vi "loadHTOutcounterFixHeader.vi"() -> ()   [LabVIEW 2012]
uses:
  <vilib>/addons/database/Connection.llb/DB Tools Open Connec (Path).vi
  <vilib>/Utility/file.llb/Read From Spreadsheet File (string).vi
  <vilib>/addons/database/Connection.llb/Conn Execute.vi
  <vilib>/addons/database/Recordset.llb/Rec Fetch Integer Data (R).vi
  <vilib>/addons/database/Recordset.llb/Rec Destroy - Connection.vi
  <vilib>/addons/database/NI_Database_API.lvlib
panel:
  out "before substring":string
  out "x > y?":bool
  out "error out":errorcluster
  in  "file (use dialog)":path=path "C:/temp/ht/MachineState/MachineState.txt"
  out "ToRunSite":string
  out "error out 2":errorcluster
  in  "input cluster":T1
  out "output cluster":T1
  out "SQLDateTime":string
  out "time stamp":timestamp
  out "SQLDateTime 2":string
  out "concatenated string":string
  out "all rows":string[][](array[string])
  out "size(s)":i32[](array[numeric])
  out "output cluster 2":T2
  in  "input cluster 2":T2
  out "before substring 5":string
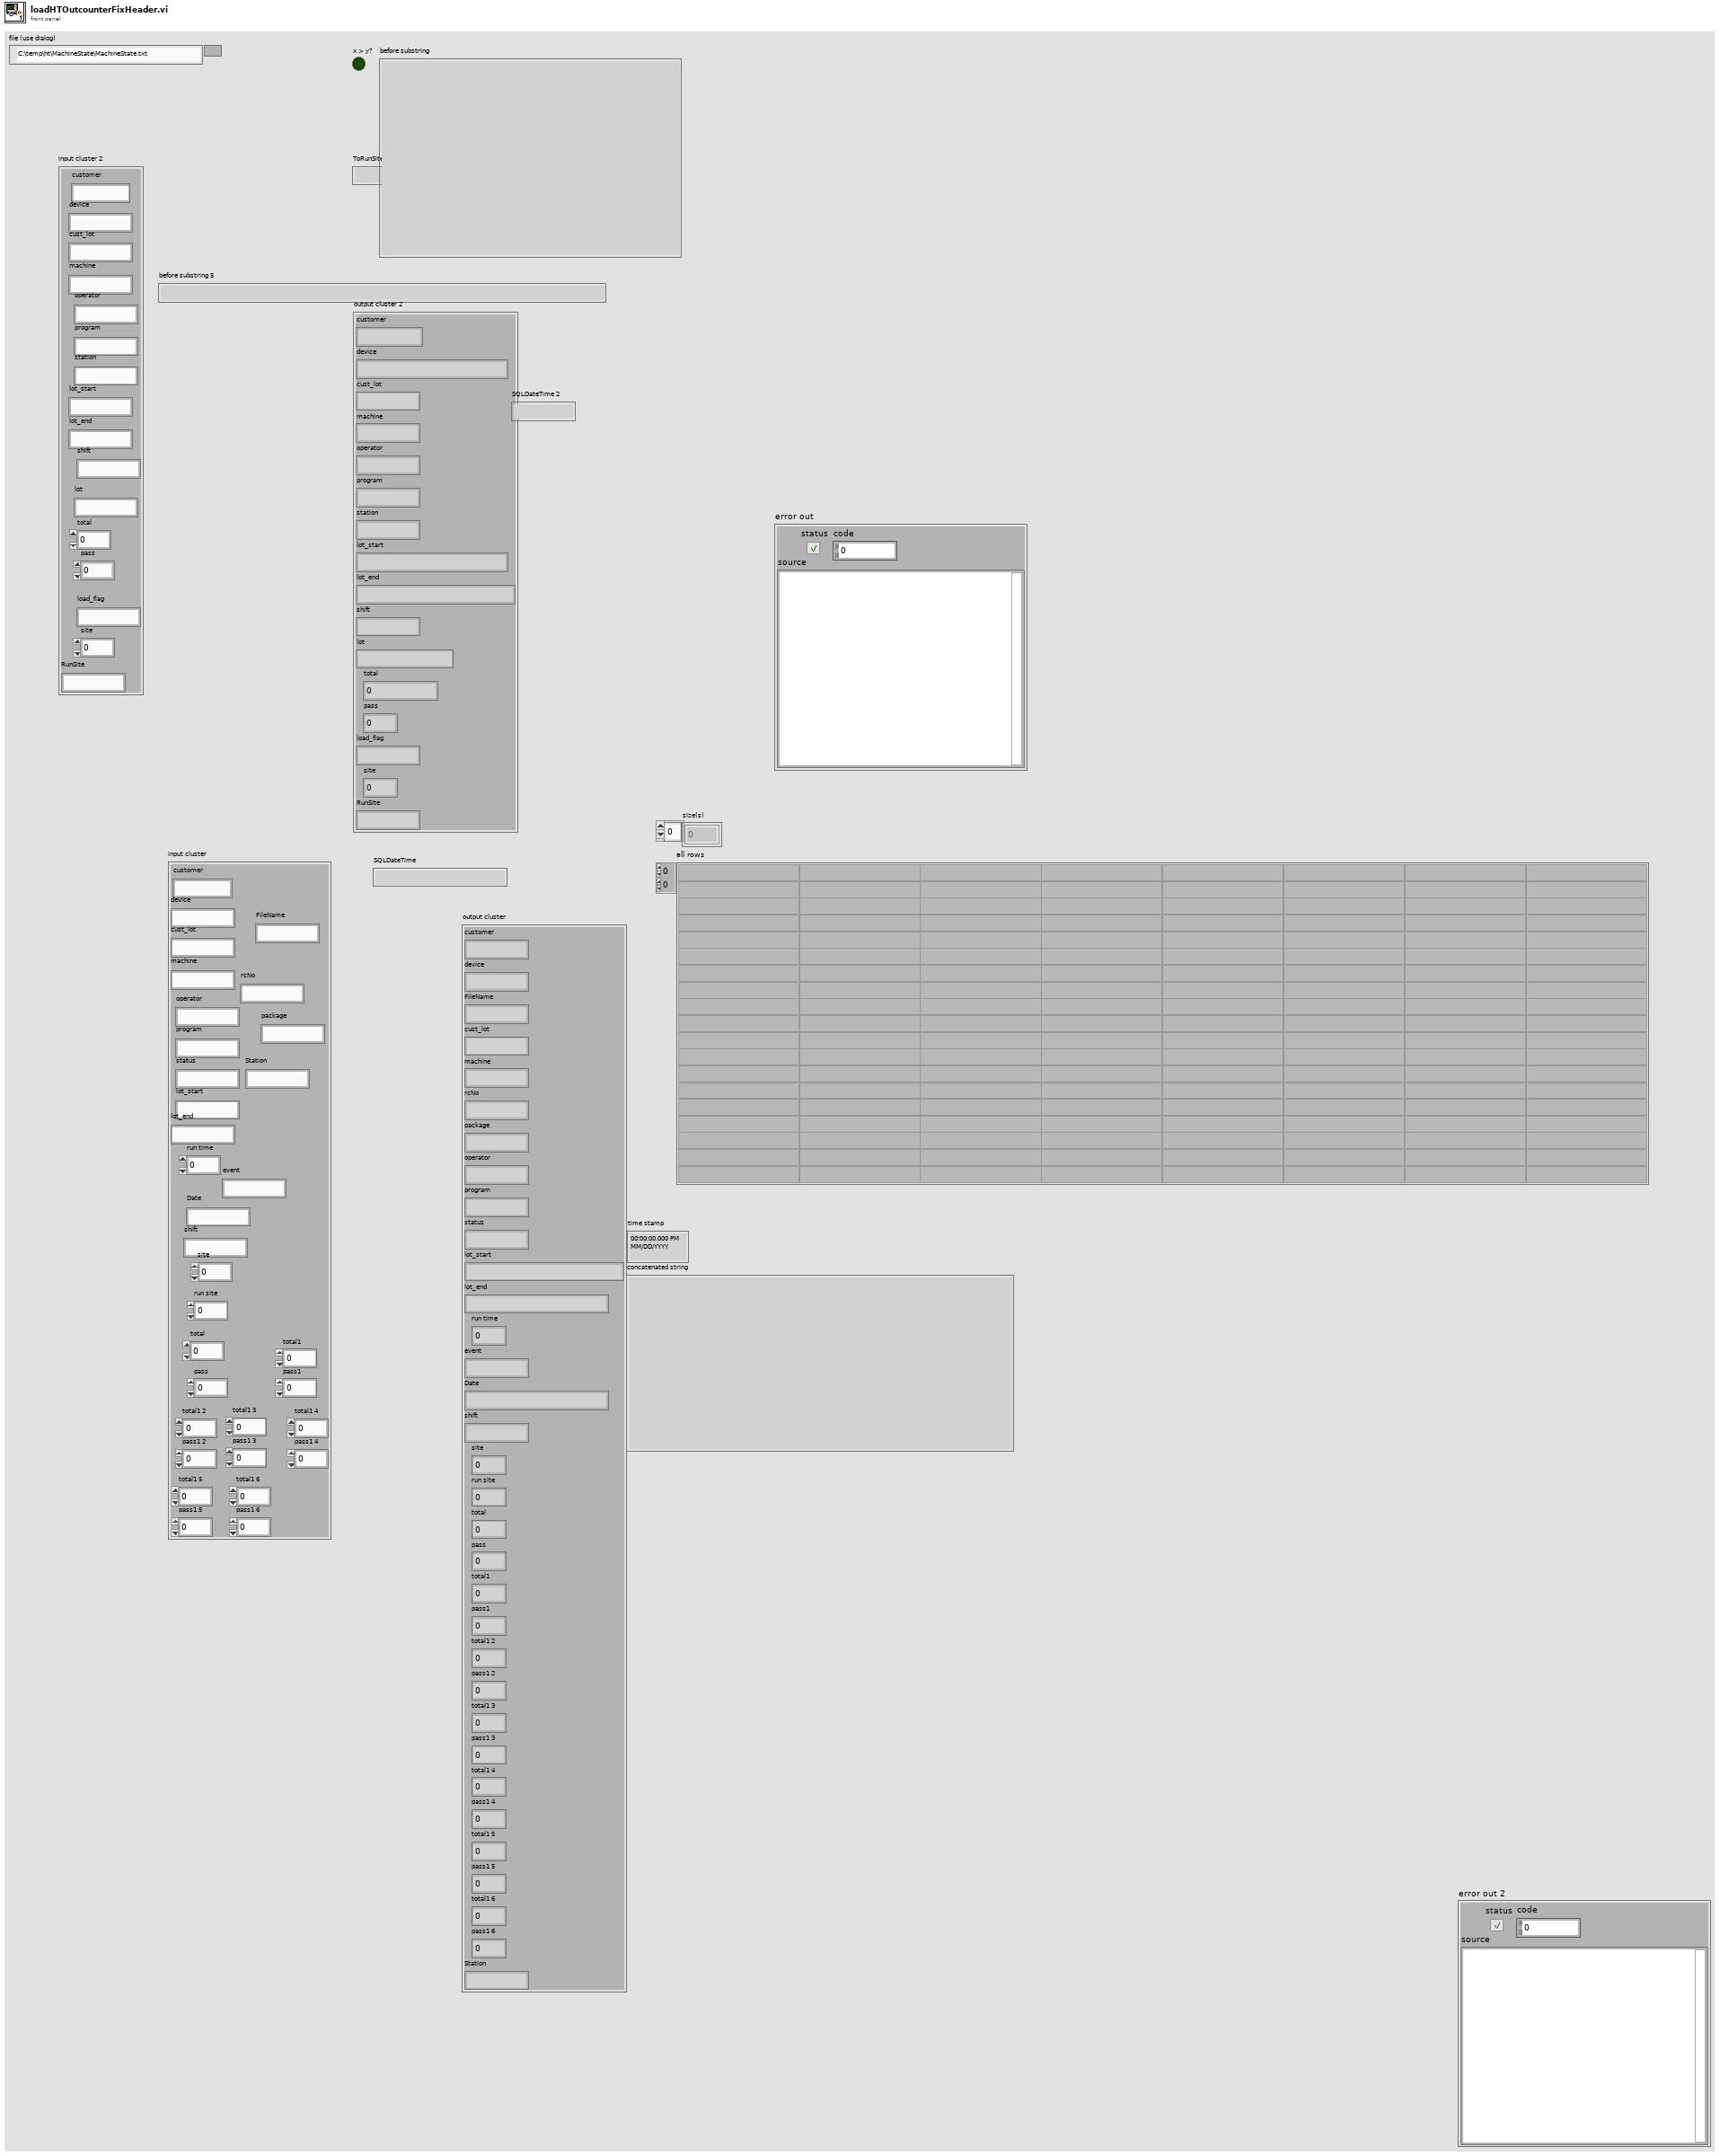
[diagram p1: front panel]
types:
  T1 = cluster{"customer":string, "device":string, "FileName":string, "cust_lot":string, "machine":string, "rcNo":string, "package":string, "operator":string, "program":string, "status":string, "lot_start":string, "lot_end":string, "run time":dbl, "event":string, "Date":string, "shift":string, "site":dbl, "run site ":dbl, "total":dbl, "pass":dbl, "total1":dbl, "pass1":dbl, "total1 2":dbl, "pass1 2":dbl, "total1 3":dbl, "pass1 3":dbl, "total1 4":dbl, "pass1 4":dbl, "total1 5":dbl, "pass1 5":dbl, "total1 6":dbl, "pass1 6":dbl, "Station":string}
  T2 = cluster{"customer":string, "device":string, "cust_lot":string, "machine":string, "operator":string, "program":string, "station":string, "lot_start":string, "lot_end":string, "shift":string, "lot":string, "total":dbl, "pass":dbl, "load_flag":string, "site":dbl, "RunSite":string}
  T3 = typedef "NI_Database_API.lvlib/Conn ObjectReference.ctl" = refnum<k1>
  T4 = typedef "NI_Database_API.lvlib/Rec ObjectReference.ctl" = refnum<k1>
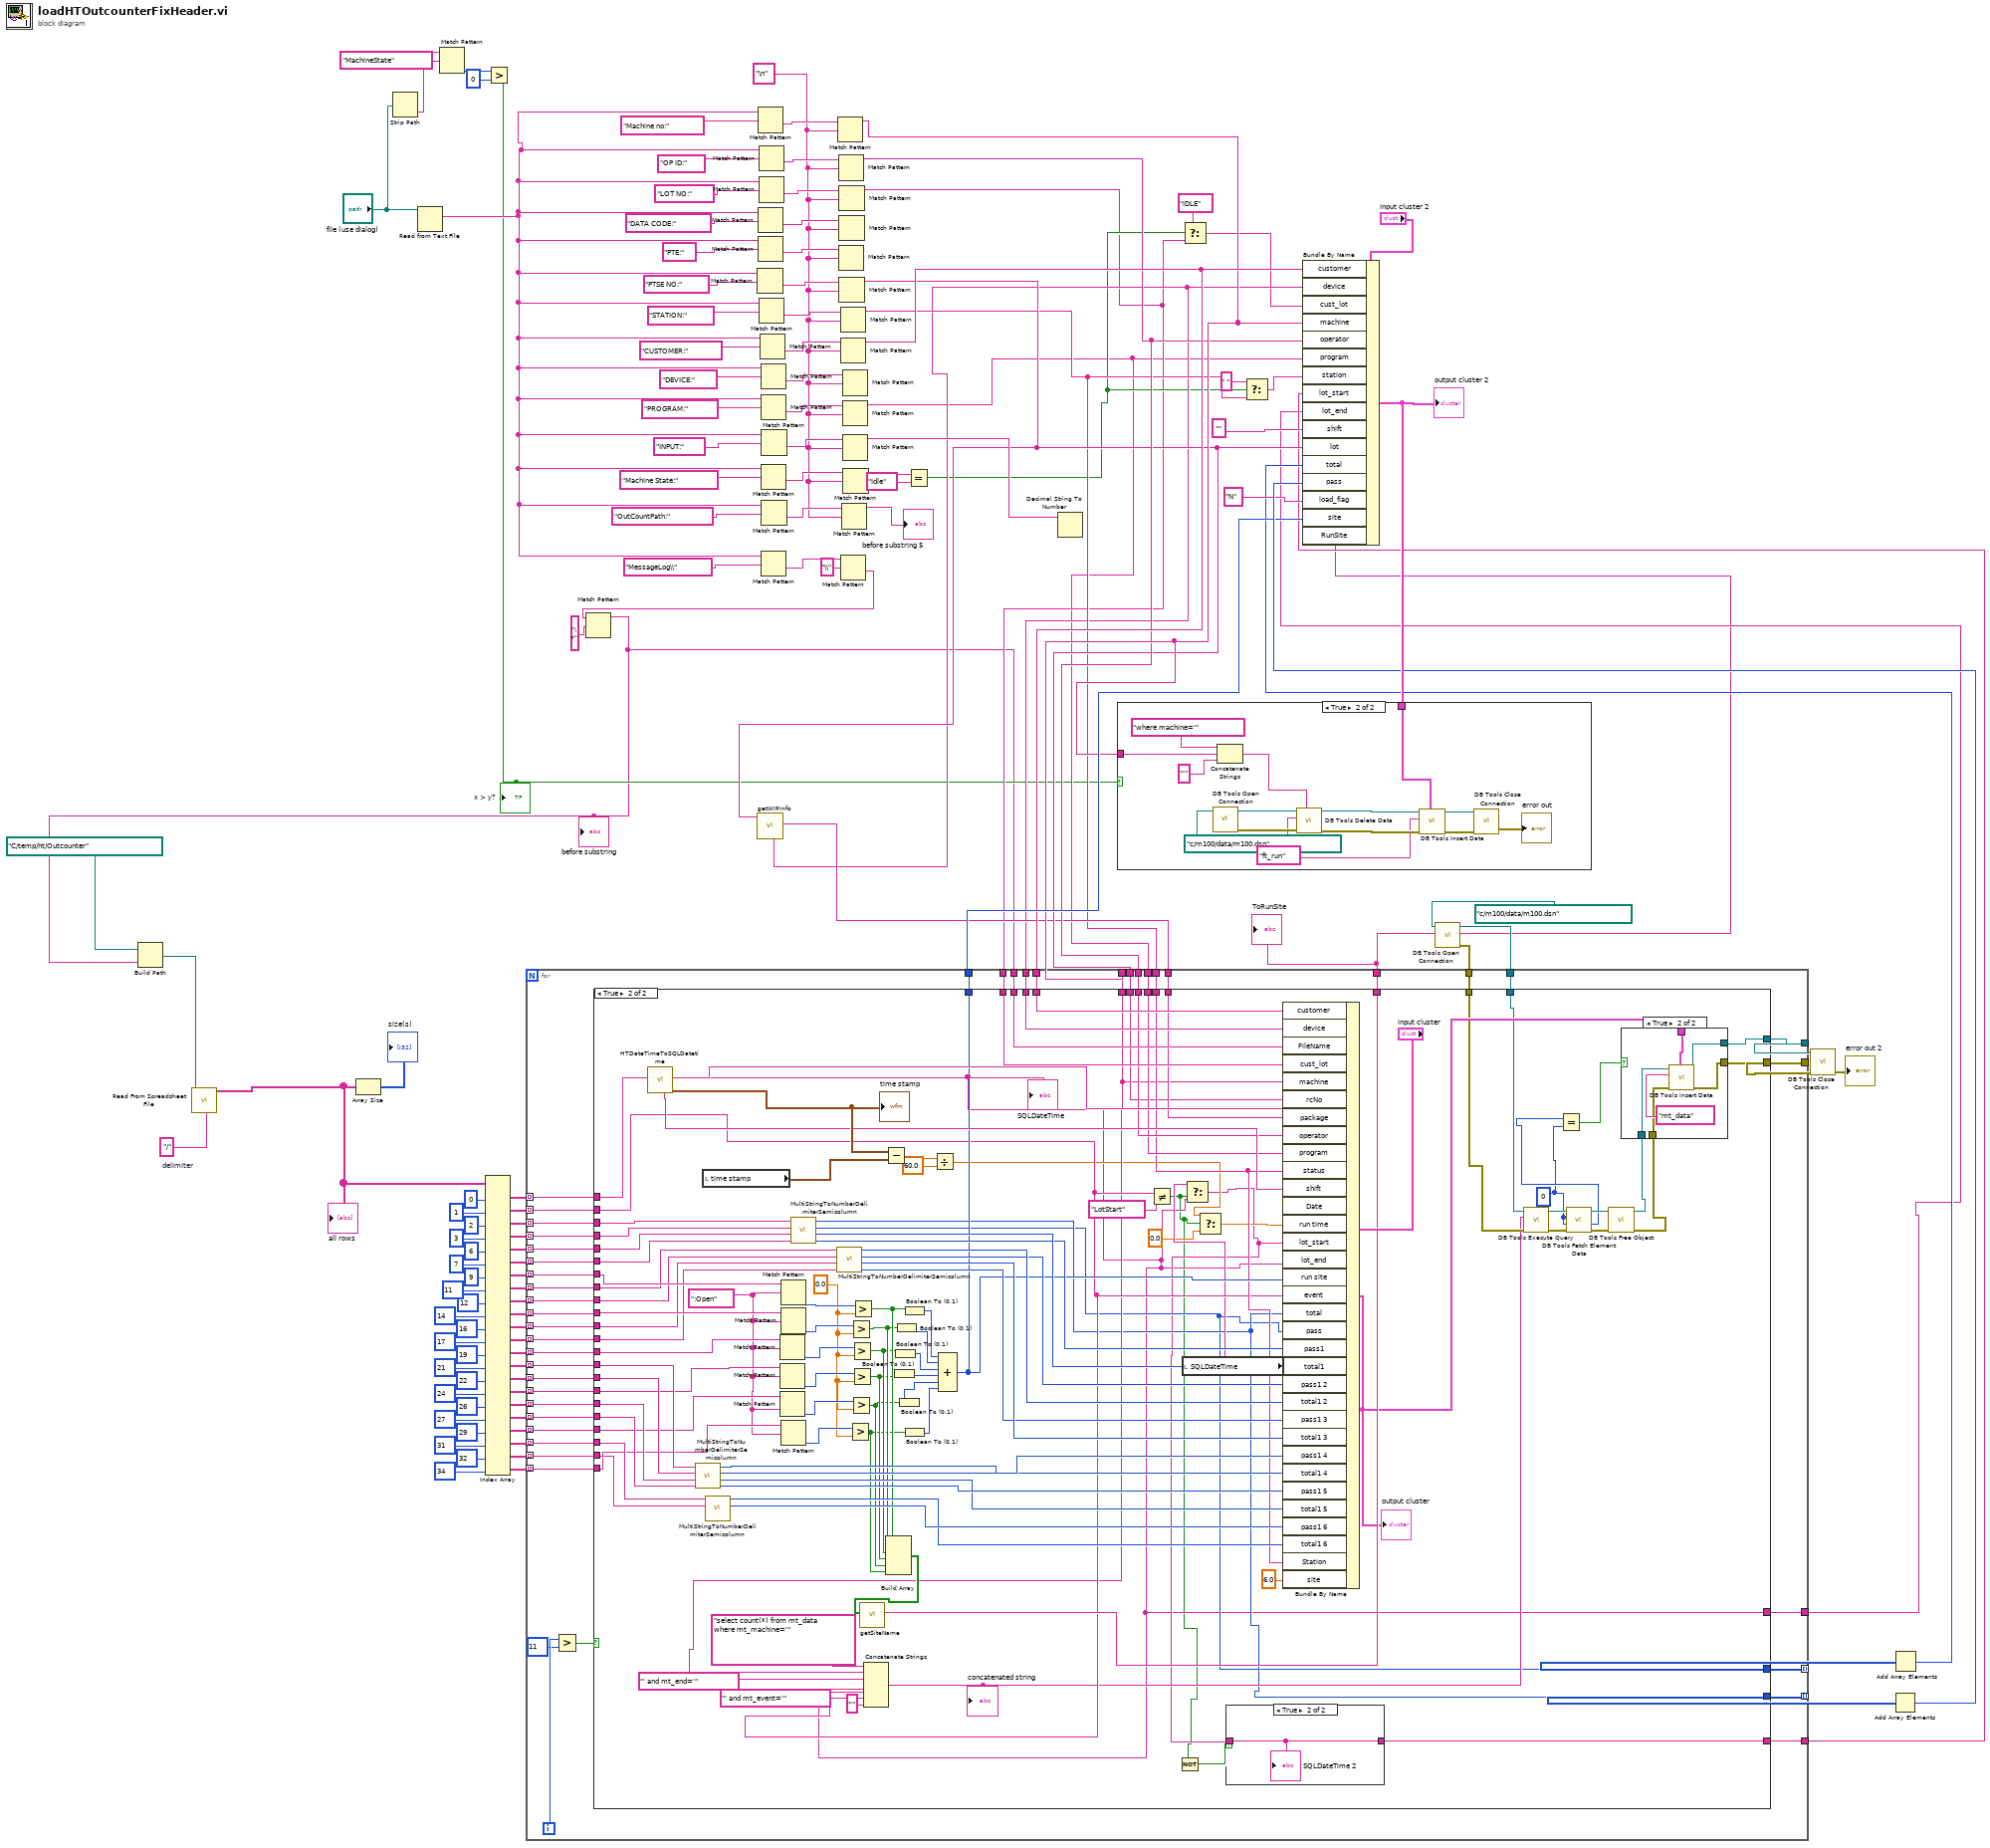
[diagram p0: block diagram]
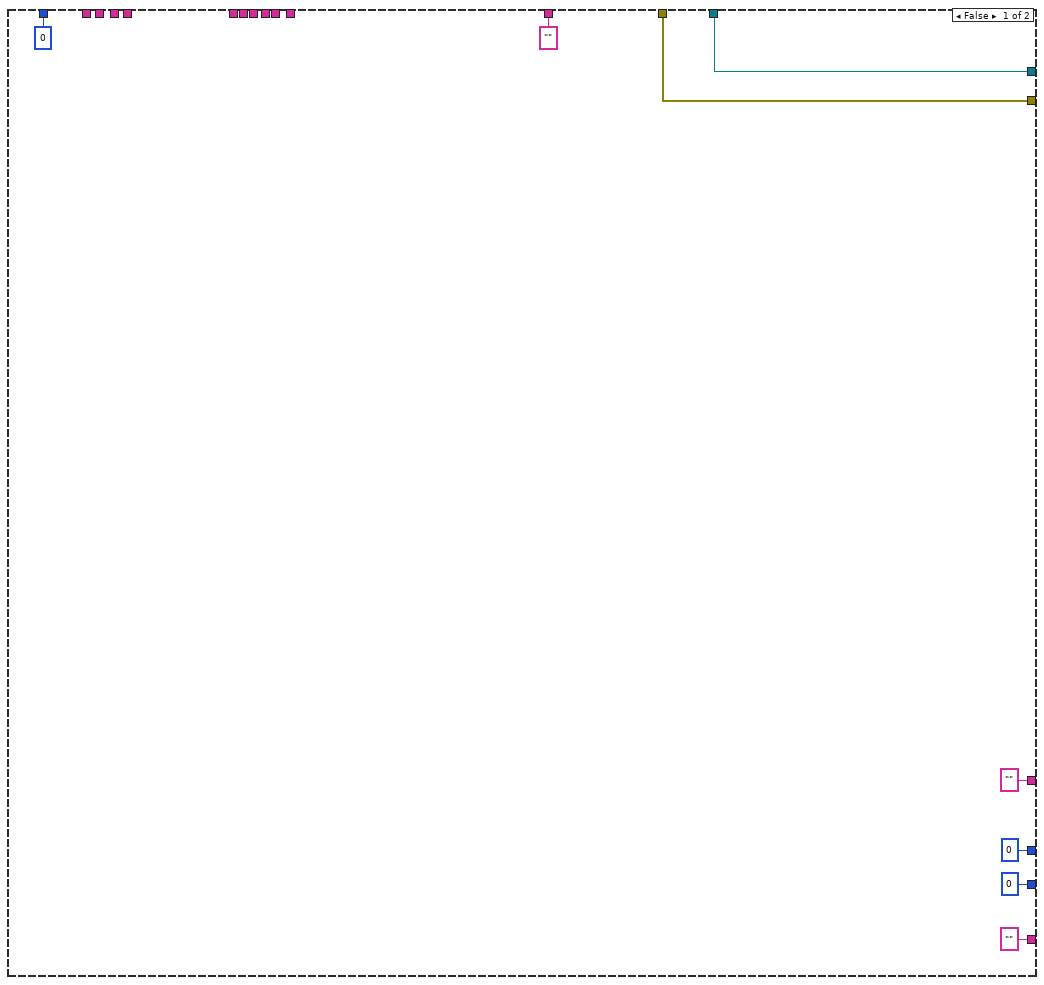
[diagram p3: hidden frame]
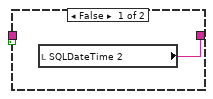
[diagram p5: hidden frame]
diagram:
  w89 = "/"  # delimiter
  w95 = "\n" ("regular expression")
  n1 = Strip Path(path="file (use dialog)") -> (name=w9:string)  [unwired: 1 out]
  n2 = Read from Text File(file (use dialog)="file (use dialog)") -> (text=w92:string)  [unwired: 3 in, 3 out]
  n3 = Match Pattern(string=w9, regular expression="MachineState") -> (offset past match=w7:i32)  [unwired: 1 in, 3 out]
  n4 = Greater?(x=w7, y=0) -> (0:w5:bool)
  "x > y?" <- w5
  n5 = Match Pattern(string=w92, regular expression="PTSE NO:") -> (after substring=w116:string)  [unwired: 1 in, 3 out]
  n6 = Match Pattern(string=w92, regular expression="Machine no:") -> (after substring=w96:string)  [unwired: 1 in, 3 out]
  n7 = Match Pattern(string=w92, regular expression="DATA CODE:") -> (after substring=w120:string)  [unwired: 1 in, 3 out]
  n8 = Match Pattern(string=w92, regular expression="PTE:") -> (after substring=w118:string)  [unwired: 1 in, 3 out]
  n9 = Match Pattern(string=w92, regular expression="OP ID:") -> (after substring=w124:string)  [unwired: 1 in, 3 out]
  n10 = Match Pattern(string=w92, regular expression="LOT NO:") -> (after substring=w122:string)  [unwired: 1 in, 3 out]
  n11 = Match Pattern(string=w92, regular expression="STATION:") -> (after substring=w103:string)  [unwired: 1 in, 3 out]
  n12 = Match Pattern(string=w92, regular expression="CUSTOMER:") -> (after substring=w114:string)  [unwired: 1 in, 3 out]
  n13 = Match Pattern(string=w92, regular expression="DEVICE:") -> (after substring=w112:string)  [unwired: 1 in, 3 out]
  n14 = Match Pattern(string=w92, regular expression="PROGRAM:") -> (after substring=w110:string)  [unwired: 1 in, 3 out]
  n15 = Match Pattern(string=w92, regular expression="Machine State:") -> (after substring=w106:string)  [unwired: 1 in, 3 out]
  n16 = Match Pattern(string=w92, regular expression="MessageLog\\") -> (after substring=w90:string)  [unwired: 1 in, 3 out]
  n17 = Match Pattern(string=w92, regular expression="INPUT:") -> (after substring=w108:string)  [unwired: 1 in, 3 out]
  n18 = Match Pattern(string=w92, regular expression="OutCountPath:") -> (after substring=w104:string)  [unwired: 1 in, 3 out]
  n19 = Match Pattern(string=w96, regular expression=w95) -> (before substring=w33:string)  [unwired: 1 in, 3 out]
  n20 = Match Pattern(string=w124, regular expression=w95) -> (before substring=w32:string)  [unwired: 1 in, 3 out]
  n21 = Match Pattern(string=w118, regular expression=w95) -> ()  [unwired: 1 in, 4 out]
  n22 = Match Pattern(string=w122, regular expression=w95) -> (before substring=w14:string)  [unwired: 1 in, 3 out]
  n23 = Match Pattern(string=w120, regular expression=w95) -> ()  [unwired: 1 in, 4 out]
  n24 = Match Pattern(string=w116, regular expression=w95) -> (before substring=w31:string)  [unwired: 1 in, 3 out]
  n25 = call "getWIPInfo.vi"("Lotno"=w31) -> ("Package"=w30:string, "Product"=w16:string)  [unwired: 4 in, 5 out]
  n26 = Match Pattern(string=w103, regular expression=w95) -> (before substring=w19:string)  [unwired: 1 in, 3 out]
  n27 = Match Pattern(string=w114, regular expression=w95) -> (before substring=w34:string)  [unwired: 1 in, 3 out]
  n28 = Match Pattern(string=w90, regular expression="\\") -> (after substring=w42:string)  [unwired: 1 in, 3 out]
  n29 = Match Pattern(string=w42, regular expression="\n") -> (before substring=w1:string)  [unwired: 1 in, 3 out]
  "before substring" <- w1
  n30 = Build Path(base path=path "C:/temp/ht/Outcounter", name or relative path=w1) -> (appended path=w3:path)
  n31 = call-poly <vilib>:"Read From Spreadsheet File.vi"("delimiter (\\t)"=w89, "file path (dialog if empty)"=w3) -> ("all rows"=w87:string[][])  [unwired: 5 in, 4 out]
  "all rows" <- w87
  n32 = Array Size(array=w87) -> (size(s)=→"size(s)":i32[])
  n33 = Index Array(array=w87, index (col) #1=0 ("disabled index (col)"), index (col) #2=1 ("index (col)"), index (col) #3=2 ("index (col)"), index (col) #4=3 ("index (col)"), index (col) #5=6 ("index (col)"), index (col) #6=7 ("index (col)"), index (col) #7=9 ("index (col)"), index (col) #8=11 ("index (col)"), index (col) #9=12 ("index (col)"), index (col) #10=14 ("index (col)"), index (col) #11=16 ("index (col)"), index (col) #12=17 ("index (col)"), index (col) #13=19 ("index (col)"), index (col) #14=21 ("index (col)"), index (col) #15=22 ("index (col)"), index (col) #16=24 ("index (col)"), index (col) #17=26 ("index (col)"), index (col) #18=27 ("index (col)"), index (col) #19=29 ("index (col)"), index (col) #20=31 ("index (col)"), index (col) #21=32 ("index (col)"), index (col) #22=34 ("index (col)")) -> (element #1=w85:string[], element #2=w83:string[], element #3=w80:string[], element #4=w79:string[], element #5=w76:string[], element #6=w75:string[], element #7=w73:string[], element #8=w70:string[], element #9=w69:string[], element #10=w67:string[], element #11=w64:string[], element #12=w63:string[], element #13=w61:string[], element #14=w58:string[], element #15=w57:string[], element #16=w55:string[], element #17=w52:string[], element #18=w51:string[], element #19=w49:string[], element #20=w46:string[], element #21=w45:string[], element #22=w43:string[])  [unwired: 22 in]
  n34 = Match Pattern(string=w104, regular expression=w95) -> (before substring=→"before substring 5":string)  [unwired: 1 in, 3 out]
  n35 = Match Pattern(string=w112, regular expression=w95) -> ()  [unwired: 1 in, 4 out]
  n36 = Match Pattern(string=w110, regular expression=w95) -> (before substring=w11:string)  [unwired: 1 in, 3 out]
  n37 = Match Pattern(string=w108, regular expression=w95) -> (before substring=w98:string)  [unwired: 1 in, 3 out]
  n38 = Match Pattern(string=w106, regular expression=w95) -> (before substring=w21:string)  [unwired: 1 in, 3 out]
  n39 = Equal?(x=w21, y="Idle") -> (x = y?=w15:bool)
  n40 = Decimal String To Number(string=w98) -> ()  [unwired: 2 in, 2 out]
  n41 = Select(t="IDLE", s=w15, f=w14) -> (s? t:f=w13:string)
  n42 = Select(t=" ", s=w15, f=w19) -> (s? t:f=w18:string)
  n43 = call-poly <vilib>:"DB Tools Open Connection.vi"("connection information"=path "c:/m100/data/m100.dsn") -> ("error out"=w27:errorcluster, "connection reference"=w28:T3)  [unwired: 7 in]
  n44 = for {
    tunnel: w85 -> [w170] mode=indexing
    tunnel: w83 -> [w136] mode=indexing
    tunnel: w80 -> [w168] mode=indexing
    tunnel: w79 -> [w167] mode=indexing
    tunnel: w76 -> [w166] mode=indexing
    tunnel: w75 -> [w165] mode=indexing
    tunnel: w73 -> [w169] mode=indexing
    tunnel: w70 -> [w164] mode=indexing
    tunnel: w69 -> [w163] mode=indexing
    tunnel: w67 -> [w162] mode=indexing
    tunnel: w64 -> [w161] mode=indexing
    tunnel: w63 -> [w160] mode=indexing
    tunnel: w61 -> [w159] mode=indexing
    tunnel: w58 -> [w158] mode=indexing
    tunnel: w57 -> [w157] mode=indexing
    tunnel: w55 -> [w156] mode=indexing
    tunnel: w52 -> [w155] mode=indexing
    tunnel: w51 -> [w154] mode=indexing
    tunnel: w49 -> [w153] mode=indexing
    tunnel: w46 -> [w152] mode=indexing
    tunnel: w45 -> [w151] mode=indexing
    tunnel: w43 -> [w150] mode=indexing
    tunnel: [w132] -> w40 mode=indexing
    tunnel: [w141] -> w38
    tunnel: [w149] -> w4
    tunnel: [w131] -> w36 mode=indexing
    tunnel: w34 -> [w148]
    tunnel: w16 -> [w147]
    tunnel: w1 -> [w146]
    tunnel: w14 -> [w145]
    tunnel: w33 -> [w133]
    tunnel: w31 -> [w137]
    tunnel: w32 -> [w144]
    tunnel: w11 -> [w143]
    tunnel: w19 -> [w138]
    tunnel: w30 -> [w142]
    tunnel: w28 -> [w135]
    tunnel: w27 -> [w134]
    tunnel: [w140] -> w25
    tunnel: [w139] -> w24
    tunnel: [w130] -> w23
    tunnel: [w129] -> w22
    i -> [w128]
    n45 = Greater?(x=w128, y=11) -> (0:w126:bool)
    n46 = case shown="True" w126 {
      tunnel: w170 -> [_ w284]
      tunnel: w169 -> [_ w283]
      tunnel: w168 -> [_ w282]
      tunnel: w167 -> [_ w281]
      tunnel: w166 -> [_ w280]
      tunnel: w165 -> [_ w279]
      tunnel: w164 -> [_ w278]
      tunnel: w163 -> [_ w277]
      tunnel: w162 -> [_ w276]
      tunnel: w161 -> [_ w275]
      tunnel: w160 -> [_ w274]
      tunnel: w159 -> [_ w273]
      tunnel: w158 -> [_ w272]
      tunnel: w157 -> [_ w271]
      tunnel: w156 -> [_ w270]
      tunnel: w155 -> [_ w269]
      tunnel: w154 -> [_ w268]
      tunnel: w153 -> [_ w267]
      tunnel: w152 -> [_ w266]
      tunnel: w151 -> [_ w265]
      tunnel: w150 -> [_ w251]
      tunnel: ["" ("String") w223] -> w149
      tunnel: w148 -> [_ w222]
      tunnel: w147 -> [_ w221]
      tunnel: w146 -> [_ w220]
      tunnel: w145 -> [_ w219]
      tunnel: w144 -> [_ w218]
      tunnel: w143 -> [_ w217]
      tunnel: w142 -> [_ w216]
      tunnel: [i16 0 w215] -> w141
      tunnel: [w172 w214] -> w140
      tunnel: [w171 w213] -> w139
      tunnel: w138 -> [_ w210]
      tunnel: w137 -> [_ w205]
      tunnel: w136 -> [_ w204]
      tunnel: w135 -> [w172 w199]
      tunnel: w134 -> [w171 w198]
      tunnel: w133 -> [_ w191]
      tunnel: [0 ("number") w188] -> w132
      tunnel: [0 ("number 2") w187] -> w131
      tunnel: ["" ("SQLDateTime") w183] -> w130
      tunnel: ["" ("SQLDateTime") w182] -> w129
      frame False {
      }
      frame True {
        w195 = 0
        w243 = 0.0 ("y")
        w250 = ":Open" ("regular expression")
        n47 = call "HTDateTimeToSQLDatetime.vi"("HTDateTime"=w284) -> ("time stamp"=w235:timestamp, "date string"=w232:string, "SQLDateTime"=w182:string, "Shift"=w231:string)  [unwired: 7 in]
        "SQLDateTime" <- w182
        "time stamp" <- w235
        n48 = call "MultiStringToNumberDelimiterSemicolumn.vi"("input string 4"=w268, "input string 3"=w269, "input string 2"=w271, "input string"=w272) -> ("number 4"=w261:i32, "number 3"=w260:i32, "number 2"=w259:i32, "number"=w258:i32)  [unwired: 4 in]
        n49 = local read "time stamp"() -> (w236:timestamp)
        n50 = call "MultiStringToNumberDelimiterSemicolumn.vi"("input string 2"=w265, "input string"=w266) -> ("number 2"=w263:i32, "number"=w262:i32)  [unwired: 6 in, 2 out]
        n51 = Match Pattern(string=w273, regular expression=w250) -> (offset past match=w247:i32)  [unwired: 1 in, 3 out]
        n52 = Match Pattern(string=w270, regular expression=w250) -> (offset past match=w246:i32)  [unwired: 1 in, 3 out]
        n53 = Match Pattern(string=w267, regular expression=w250) -> (offset past match=w245:i32)  [unwired: 1 in, 3 out]
        n54 = Match Pattern(string=w283, regular expression=w250) -> (offset past match=w249:i32)  [unwired: 1 in, 3 out]
        n55 = Match Pattern(string=w276, regular expression=w250) -> (offset past match=w248:i32)  [unwired: 1 in, 3 out]
        n56 = Match Pattern(string=w251, regular expression=w250) -> (offset past match=w244:i32)  [unwired: 1 in, 3 out]
        n57 = call "MultiStringToNumberDelimiterSemicolumn.vi"("input string 4"=w279, "input string 3"=w280, "input string 2"=w281, "input string"=w282) -> ("number 4"=w252:i32, "number 3"=w253:i32, "number 2"=w187:i32, "number"=w188:i32)  [unwired: 4 in]
        n58 = call "MultiStringToNumberDelimiterSemicolumn.vi"("input string 4"=w274, "input string 3"=w275, "input string 2"=w277, "input string"=w278) -> ("number 4"=w256:i32, "number 3"=w257:i32, "number 2"=w254:i32, "number"=w255:i32)  [unwired: 4 in]
        n59 = Greater?(x=w244, y=w243) -> (0:w225:bool)
        n60 = Greater?(x=w248, y=w243) -> (0:w229:bool)
        n61 = Greater?(x=w245, y=w243) -> (0:w226:bool)
        n62 = Greater?(x=w247, y=w243) -> (0:w228:bool)
        n63 = Greater?(x=w246, y=w243) -> (0:w227:bool)
        n64 = Greater?(x=w249, y=w243) -> (0:w230:bool)
        n65 = Concatenate Strings("select count(*) from mt_data where mt_machine='" ("string"), w191, "' and mt_end='" ("string"), w182, "' and mt_event='" ("string"), w204, "'" ("string")) -> (w197:string)
        "concatenated string" <- w197
        n66 = Subtract(x=w235, y=w236) -> (x-y=w234:dbl)
        n67 = Build Array(w230, w229, w228, w227, w226, w225) -> (w224:bool[])
        n68 = call "getSiteName.vi"("Array"=w224) -> ("String"=w223:string)  [unwired: 10 in]
        n69 = Boolean To (0,1)(Boolean=w227) -> (0, 1=w239:i16)
        n70 = Boolean To (0,1)(Boolean=w228) -> (0, 1=w240:i16)
        n71 = Boolean To (0,1)(Boolean=w229) -> (0, 1=w241:i16)
        n72 = Boolean To (0,1)(Boolean=w226) -> (0, 1=w238:i16)
        n73 = Boolean To (0,1)(Boolean=w230) -> (0, 1=w242:i16)
        n74 = Boolean To (0,1)(Boolean=w225) -> (0, 1=w237:i16)
        n75 = Divide(x=w234, y=60.0) -> (x/y=w186:dbl)
        n76 = Compound Arithmetic op=ADD(w242, w241, w240, w239, w238, w237) -> (w215:i16)
        n77 = Not Equal?(x=w204, y="LotStart") -> (x != y?=w180:bool)
        n78 = Not(x=w180) -> (.not. x?=w179:bool)
        n79 = local read "SQLDateTime"() -> (w189:string)
        n80 = Select(t=w189, s=w180, f=w182) -> (s? t:f=w184:string)
        n81 = Select(t=w186, s=w180, f=0.0 ("t")) -> (s? t:f=w190:dbl)
        n82 = case shown="True" w179 {
          tunnel: w184 -> [_ w294]
          tunnel: [w293 w294] -> w183
          frame False {
            n83 = local read "SQLDateTime 2"() -> (w293:string)
          }
          frame True {
            "SQLDateTime 2" <- w294
          }
        }
        n84 = Bundle By Name(cluster="input cluster", "customer"=w222, "device"=w221, "FileName"=w220, "cust_lot"=w219, "machine"=w191, "rcNo"=w205, "package"=w216, "operator"=w218, "program"=w217, "status"=w210, "shift"=w231, "Date"=w232, "run time"=w190, "lot_start"=w184, "lot_end"=w182, "run site"=w215, "event"=w204, "total"=w188, "pass"=w187, "pass1"=w252, "total1"=w253, "pass1 2"=w254, "total1 2"=w255, "pass1 3"=w256, "total1 3"=w257, "pass1 4"=w259, "total1 4"=w258, "pass1 5"=w261, "total1 5"=w260, "pass1 6"=w263, "total1 6"=w262, "Station"=w210, "site"=6.0) -> (w212:T1)
        "output cluster" <- w212
        n85 = call-poly <vilib>:"DB Tools Execute Query.vi"("error in (no error)"=w198, "SQL query"=w197, "connection reference"=w199) -> ("error out"=w203:errorcluster, "recordset reference"=w202:T4)  [unwired: 5 in]
        n86 = call-poly <vilib>:"DB Tools Fetch Element Data.vi"("error in (no error)"=w203, "type"=w195, "column index"=w195, "recordset reference"=w202) -> ("error out"=w201:errorcluster, "data"=w196:i32, "recordset reference out"=w200:T4)  [unwired: 3 in]
        n87 = Equal?(x=w196, y=w195) -> (x = y?=w194:bool)
        n88 = call-poly <vilib>:"DB Tools Free Object.vi"("error in (no error)"=w201, "recordset reference"=w200) -> ("error out"=w192:errorcluster, "connection reference"=w193:T3)  [unwired: 8 in]
        n89 = case shown="True" w194 {
          tunnel: [w286 w292] -> w214
          tunnel: [w285 w291] -> w213
          tunnel: w212 -> [_ w289]
          tunnel: w193 -> [w286 w288]
          tunnel: w192 -> [w285 w287]
          frame False {
          }
          frame True {
            n90 = call <vilib>:"DB Tools Insert Data.vi"("data"=w289, "error in (no error)"=w287, "table"="mt_data", "connection reference"=w288) -> ("error out"=w291:errorcluster, "connection reference out"=w292:T3)  [unwired: 6 in]
          }
        }
      }
    }
  }
  "ToRunSite" <- w4
  n91 = call <vilib>:"DB Tools Close Connection.vi"("error in (no error)"=w24, "connection reference"=w25) -> ("error out"=→"error out 2":errorcluster)  [unwired: 5 in]
  n92 = Add Array Elements(numeric array=w40) -> (sum=w39:i32)
  n93 = Add Array Elements(numeric array=w36) -> (sum=w35:i32)
  n94 = Bundle By Name(cluster="input cluster 2", "customer"=w34, "device"=w16, "cust_lot"=w13, "machine"=w33, "operator"=w32, "program"=w11, "station"=w18, "lot_start"=w23, "lot_end"=w22, "shift"="" ("lot_end"), "lot"=w31, "total"=w35, "pass"=w39, "load_flag"="N", "site"=w38, "RunSite"=w4) -> (w94:T2)
  "output cluster 2" <- w94
  n95 = case shown="True" w5 {
    tunnel: w94 -> [_ w299]
    tunnel: w33 -> [_ w297]
    frame False {
    }
    frame True {
      w298 = "ft_run" ("table")
      n96 = call-poly <vilib>:"DB Tools Open Connection.vi"("connection information"=path "c:/m100/data/m100.dsn") -> ("error out"=w307:errorcluster, "connection reference"=w308:T3)  [unwired: 7 in]
      n97 = Concatenate Strings("where machine='" ("string"), w297, "'" ("string")) -> (w303:string)
      n98 = call <vilib>:"DB Tools Delete Data.vi"("condition"=w303, "error in (no error)"=w307, "table"=w298, "connection reference"=w308) -> ("error out"=w300:errorcluster, "connection reference out"=w301:T3)  [unwired: 6 in]
      n99 = call <vilib>:"DB Tools Insert Data.vi"("data"=w299, "error in (no error)"=w300, "table"=w298, "connection reference"=w301) -> ("error out"=w295:errorcluster, "connection reference out"=w296:T3)  [unwired: 6 in]
      n100 = call <vilib>:"DB Tools Close Connection.vi"("error in (no error)"=w295, "connection reference"=w296) -> ("error out"=→"error out":errorcluster)  [unwired: 5 in]
    }
  }
